vi "Agilent 2000 3000 X-Series Acquire Waveform Continuously.vi"() -> ()   [LabVIEW 2015]
doc: "This example shows how to use autosetup and acquire a waveform continuously on a single channel.\n\n<B>Note:</B> In this example, each record is acquired independently and not as a continuous stream of data."
uses:
  <instrlib>/Agilent 2000 3000 X-Series/Agilent 2000 3000 X-Series.lvlib
panel:
  in  "Source Channel (0: Channel 1)":i32(ring) items=["Channel 1"=0, "Channel 2"=1, "Channel 3"=2, "Channel 4"=3, "Digital Bus Low"=9, "Digital Bus High"=10]
  in  "Maximum Time (10000 ms)":u32=10000
  in  "stop":bool
  in  "Probe Attenuation (10.0)":dbl=10.0
  out "Waveform Data":waveform(dbl)(graph)
  in  "VISA resource name":refnum<visa-resource-name>
  # "(c) 2011-2016 National Instruments.  ALL RIGHTS RESERVED."
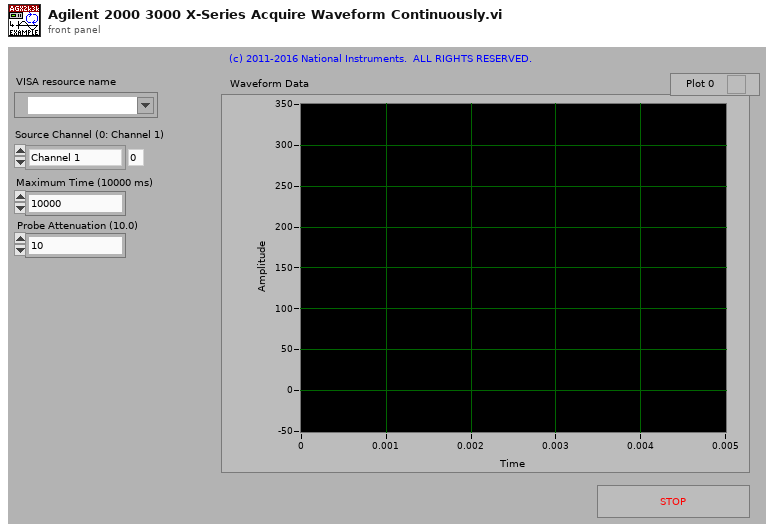
[diagram p1: front panel]
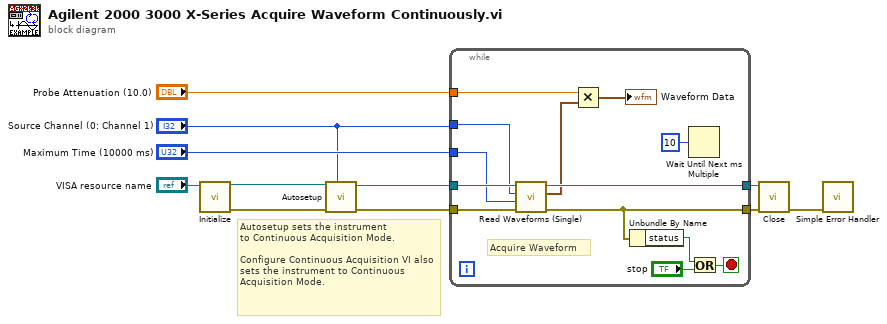
[diagram p0: block diagram]
diagram:
  # "Autosetup sets the instrument\nto Continuous Acquisition Mode.\n\nConfigure Continuous Acquisition VI also sets the instrument to Continuous Acquisition Mode."
  n1 = call <instrlib>:"Initialize.vi"("VISA resource name"="VISA resource name") -> ("error out"=w7:errorcluster, "VISA resource name out"=w6:refnum<visa-resource-name>)  [unwired: 4 in, 5 out]
  n2 = call <instrlib>:"Autosetup.vi"("Auto Scale Source (0: Channel 1)"="Source Channel (0: Channel 1)", "error in (no error)"=w7, "VISA resource name"=w6) -> ("error out"=w3:errorcluster, "VISA resource name out"=w4:refnum<visa-resource-name>)  [unwired: 3 in, 4 out]
  n3 = while {
    tunnel: w4 -> [w15]
    tunnel: w3 -> [w14]
    tunnel: [w18] -> w10
    tunnel: [w17] -> w9
    tunnel: "Probe Attenuation (10.0)" -> [w24]
    tunnel: "Maximum Time (10000 ms)" -> [w13]
    tunnel: "Source Channel (0: Channel 1)" -> [w12]
    stop <- w21 stop-if-true
    # "Acquire Waveform"
    n4 = call <instrlib>:"Read Waveforms (Single).vi"("error in (no error)"=w14, "Timeout (10000 ms)"=w13, "Source Channel (0: Channel 1)"=w12, "VISA resource name"=w15) -> ("error out"=w17:errorcluster, "Waveform Data"=w16:waveform(dbl), "VISA resource name out"=w18:refnum<visa-resource-name>)  [unwired: 1 in, 4 out]
    n5 = Multiply(x=w24, y=w16) -> (x*y=→"Waveform Data":waveform(dbl))
    n6 = Unbundle By Name(w17) -> ("status"=w20:bool)
    n7 = Wait Until Next ms Multiple(millisecond multiple=u32 10) -> ()  [unwired: 1 out]
    n8 = Or(x=w20, y="stop") -> (x .or. y?=w21:bool)
  }
  n9 = call <instrlib>:"Close.vi"("error in (no error)"=w9, "VISA resource name"=w10) -> ("error out"=w11:errorcluster)  [unwired: 9 out]
  n10 = call <vilib>:"Simple Error Handler.vi"("error in (no error)"=w11) -> ()  [unwired: 1 in, 8 out]
